vi "Check Data Model1.vi"(8 "error in (no error)":errorcluster, 11 "device data model in":refnum<class "Standard Data Model1.lvclass">) -> (0 "error out":errorcluster, 3 "device data model out":refnum<class "Standard Data Model1.lvclass">)   [LabVIEW 2019, in "NI_modbus_upd.lvlib" / "Standard Data Model1.lvclass"]
doc: "This VI ensures that the data model has at least 65,535 values of every type. This is required for certain modbus function codes."
uses:
  Standard Data Model1.lvclass
  Standard Data Model1.lvclass/Standard Data Model1.ctl
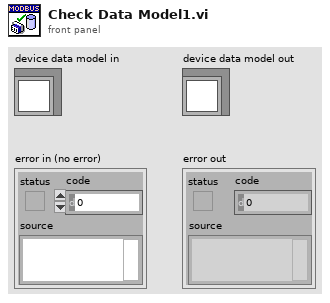
[diagram p1: front panel]
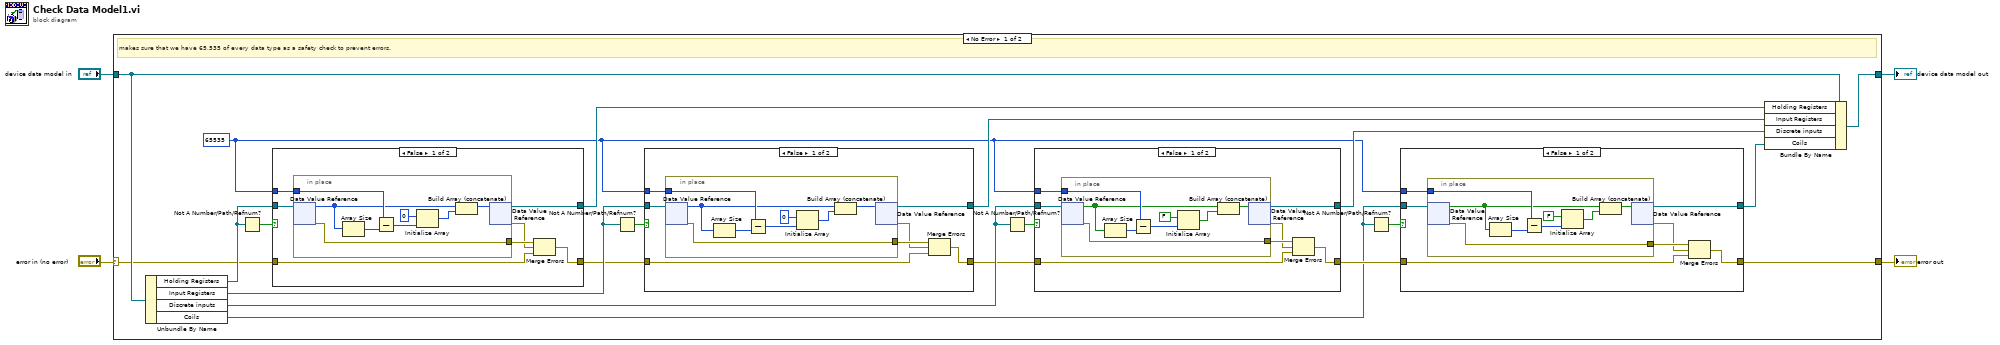
[diagram p0: block diagram]
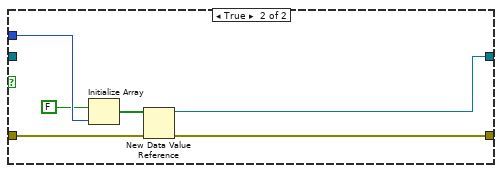
[diagram p2: hidden frame]
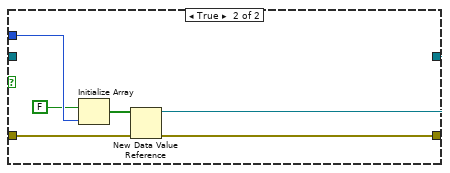
[diagram p3: hidden frame]
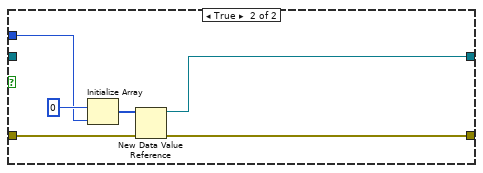
[diagram p4: hidden frame]
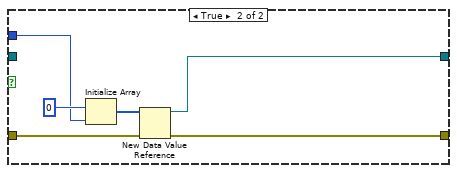
[diagram p5: hidden frame]
diagram:
  n1 = case shown="No Error" "error in (no error)" {
    selector: "error in (no error)" -> [w5 w110]
    tunnel: "device data model in" -> [w19 w109]
    tunnel: [w18 w109] -> w3
    tunnel: [w9 w110] -> w2
    frame No Error {
      w6 = u16 65535 ("x")
      # "makes sure that we have 65,535 of every data type as a safety check to prevent errors."
      n2 = Unbundle By Name(w19) -> ("Holding Registers"=w23:refnum<data-value>, "Input Registers"=w21:refnum<data-value>, "Discrete inputs"=w14:refnum<data-value>, "Coils"=w7:refnum<data-value>)
      n3 = Not A Number/Path/Refnum?(number/path/refnum=w23) -> (NaN/Path/Refnum?=w24:bool)
      n4 = case shown="False" w24 {
        tunnel: w5 -> [w88 w107]
        tunnel: [w92 w105] -> w17
        tunnel: [w93 w104] -> w20
        tunnel: w23 -> [w94 _]
        tunnel: w6 -> [w91 w103]
        frame False {
          n5 = in-place {
            in-place-border: w91 -> [w102]
            in-place-border: [w95] -> w90
            n6 = in-place-dvr #1(w94) -> (w98:u16[], w95:errorcluster)
            n7 = Array Size(array=w98) -> (size(s)=w101:i32)
            n8 = Subtract(x=w102, y=w101) -> (x-y=w100:i32)
            n9 = Initialize Array(u16 0 ("element"), w100) -> (w97:u16[])
            n10 = Build Array (concatenate)(w98, w97) -> (w96:u16[])
            n11 = in-place-dvr #1(w96) -> (w92:refnum<data-value>, w89:errorcluster)
          }
          n12 = Merge Errors(w90, w89, w88) -> (w93:errorcluster)
        }
        frame True {
          n13 = Initialize Array(u16 0 ("element"), w103) -> (w106:u16[])
          n14 = New Data Value Reference(data value=w106, error in=w107) -> (data value reference=w105:refnum<data-value>, error out=w104:errorcluster)
        }
      }
      n15 = Not A Number/Path/Refnum?(number/path/refnum=w21) -> (NaN/Path/Refnum?=w22:bool)
      n16 = case shown="False" w22 {
        tunnel: w20 -> [w67 w86]
        tunnel: [w71 w84] -> w16
        tunnel: [w72 w83] -> w12
        tunnel: w21 -> [w73 _]
        tunnel: w6 -> [w70 w82]
        frame False {
          n17 = in-place {
            in-place-border: w70 -> [w81]
            in-place-border: [w74] -> w69
            n18 = in-place-dvr #2(w73) -> (w77:u16[], w74:errorcluster)
            n19 = Array Size(array=w77) -> (size(s)=w80:i32)
            n20 = Subtract(x=w81, y=w80) -> (x-y=w79:i32)
            n21 = Initialize Array(u16 0 ("element"), w79) -> (w76:u16[])
            n22 = Build Array (concatenate)(w77, w76) -> (w75:u16[])
            n23 = in-place-dvr #2(w75) -> (w71:refnum<data-value>, w68:errorcluster)
          }
          n24 = Merge Errors(w69, w68, w67) -> (w72:errorcluster)
        }
        frame True {
          n25 = Initialize Array(u16 0 ("element"), w82) -> (w85:u16[])
          n26 = New Data Value Reference(data value=w85, error in=w86) -> (data value reference=w84:refnum<data-value>, error out=w83:errorcluster)
        }
      }
      n27 = Not A Number/Path/Refnum?(number/path/refnum=w14) -> (NaN/Path/Refnum?=w15:bool)
      n28 = case shown="False" w15 {
        tunnel: w12 -> [w48 w66]
        tunnel: [w50 w61] -> w13
        tunnel: [w51 w64] -> w8
        tunnel: w14 -> [w52 _]
        tunnel: w6 -> [w49 w63]
        frame False {
          n29 = in-place {
            in-place-border: w49 -> [w60]
            in-place-border: [w53] -> w47
            n30 = in-place-dvr #3(w52) -> (w56:bool[], w53:errorcluster)
            n31 = Array Size(array=w56) -> (size(s)=w59:i32)
            n32 = Subtract(x=w60, y=w59) -> (x-y=w58:i32)
            n33 = Initialize Array(FALSE, w58) -> (w55:bool[])
            n34 = Build Array (concatenate)(w56, w55) -> (w54:bool[])
            n35 = in-place-dvr #3(w54) -> (w50:refnum<data-value>, w46:errorcluster)
          }
          n36 = Merge Errors(w47, w46, w48) -> (w51:errorcluster)
        }
        frame True {
          n37 = Initialize Array(FALSE, w63) -> (w65:bool[])
          n38 = New Data Value Reference(data value=w65, error in=w66) -> (data value reference=w61:refnum<data-value>, error out=w64:errorcluster)
        }
      }
      n39 = Not A Number/Path/Refnum?(number/path/refnum=w7) -> (NaN/Path/Refnum?=w11:bool)
      n40 = case shown="False" w11 {
        tunnel: w8 -> [w26 w45]
        tunnel: [w29 w41] -> w10
        tunnel: [w30 w43] -> w9
        tunnel: w7 -> [w31 _]
        tunnel: w6 -> [w28 w42]
        frame False {
          n41 = in-place {
            in-place-border: w28 -> [w39]
            in-place-border: [w32] -> w27
            n42 = in-place-dvr #4(w31) -> (w35:bool[], w32:errorcluster)
            n43 = Array Size(array=w35) -> (size(s)=w38:i32)
            n44 = Subtract(x=w39, y=w38) -> (x-y=w37:i32)
            n45 = Initialize Array(FALSE, w37) -> (w34:bool[])
            n46 = Build Array (concatenate)(w35, w34) -> (w33:bool[])
            n47 = in-place-dvr #4(w33) -> (w29:refnum<data-value>, w25:errorcluster)
          }
          n48 = Merge Errors(w27, w25, w26) -> (w30:errorcluster)
        }
        frame True {
          n49 = Initialize Array(FALSE, w42) -> (w44:bool[])
          n50 = New Data Value Reference(data value=w44, error in=w45) -> (data value reference=w41:refnum<data-value>, error out=w43:errorcluster)
        }
      }
      n51 = Bundle By Name(cluster=w19, "Holding Registers"=w17, "Input Registers"=w16, "Discrete inputs"=w13, "Coils"=w10) -> (w18:refnum<class "Standard Data Model1.lvclass">)
    }
    frame Error {
    }
  }
  "error out" <- w2
  "device data model out" <- w3
